vi "camera info.vi"(8 "Disc Number":string, 10 "Camera Name":T1="cam5") -> ()   [LabVIEW 2019]
uses:
  <vilib>/userDefined/High Color/IMAQdx.ctl
  <vilib>/vision/driver/NI_Vision_Acquisition_Software.lvlib
  <resource>/objmgr/imaqdx.rc
panel:
  in  "Close":bool
  out "String":string
  out "Temperature State":string
  out "error out":errorcluster
  out "Gain Raw":u32
  out "Exposure Time":u32
  out "Temperature":dbl
  in  "error in":errorcluster
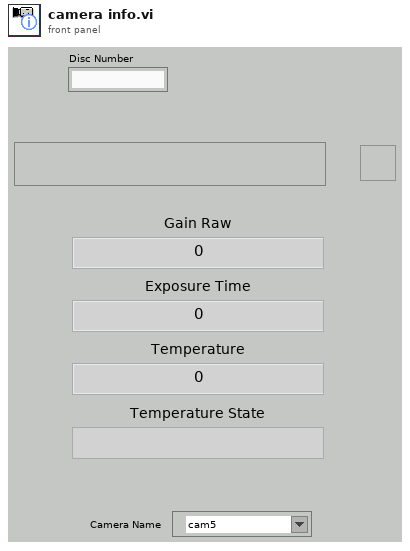
[diagram p1: front panel]
types:
  T1 = typedef "IMAQdx.ctl" = refnum<k21>
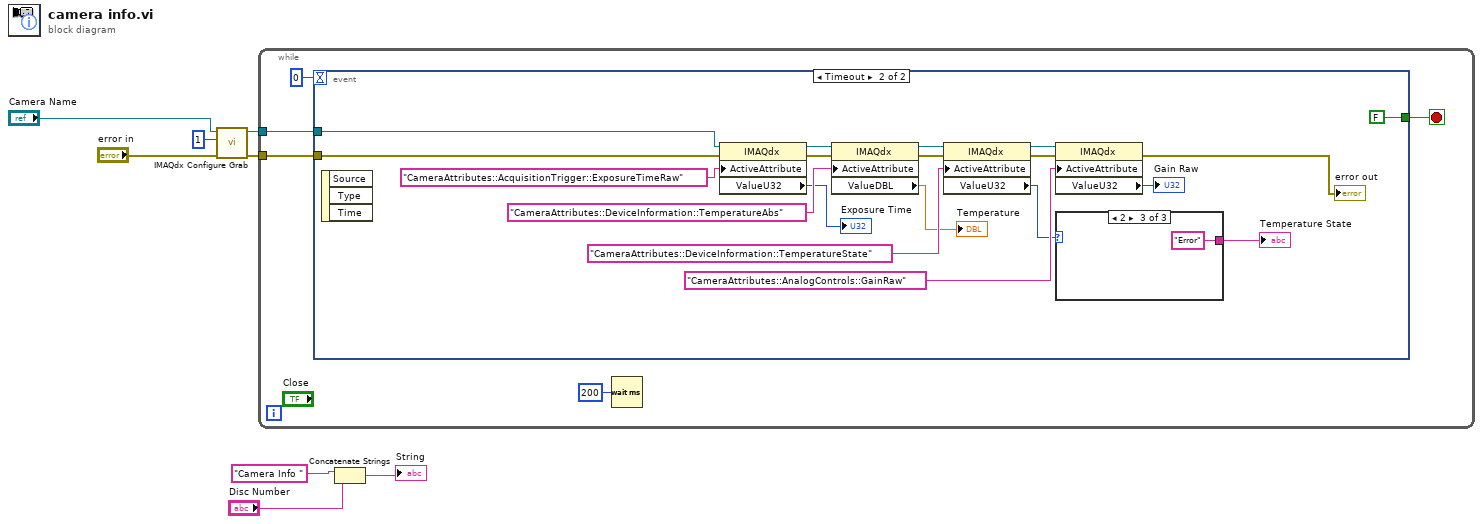
[diagram p0: block diagram]
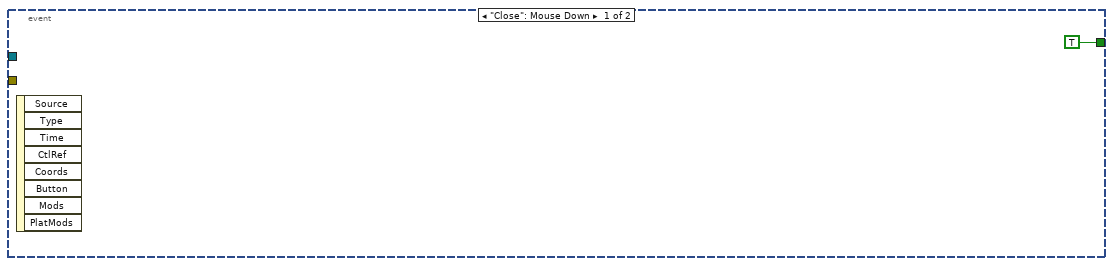
[diagram p2: hidden frame]
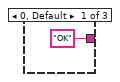
[diagram p3: hidden frame]
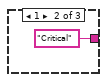
[diagram p4: hidden frame]
diagram:
  n1 = call <vilib>:"IMAQdx Configure Grab.vi"("error in"="error in", "Number of Buffers"=u32 1, "Session In"="Camera Name") -> ("error out"=w6:errorcluster, "Session Out"=w7:T1)  [unwired: 7 in]
  n2 = while {
    tunnel: w7 -> [w13]
    tunnel: w6 -> [w12]
    stop <- w10 stop-if-true
    n3 = event shown="[1] Timeout" {
      selector: _ -> [_ _]
      dyn-events: _ -> [_ _]
      timeout: 0 -> [_ _]
      tunnel: w13 -> [_ w33]
      tunnel: w12 -> [_ w32]
      tunnel: [TRUE FALSE] -> w10
      event "Close": Mouse Down {
        n4 = event-data() -> ()  [unwired: 1 in, 8 out]
      }
      event Timeout {
        n5 = event-data() -> ()  [unwired: 1 in, 3 out]
        n6 = property class="IMAQdx"(reference=w33, error in=w32, "ActiveAttribute"="CameraAttributes::AcquisitionTrigger::ExposureTimeRaw") -> (reference out=w28:T1, error out=w29:errorcluster, "ValueU32"=→"Exposure Time":u32)
        n7 = property class="IMAQdx"(reference=w28, error in=w29, "ActiveAttribute"="CameraAttributes::DeviceInformation::TemperatureAbs") -> (reference out=w27:T1, error out=w26:errorcluster, "ValueDBL"=→"Temperature":dbl)
        n8 = property class="IMAQdx"(reference=w27, error in=w26, "ActiveAttribute"="CameraAttributes::DeviceInformation::TemperatureState") -> (reference out=w24:T1, error out=w23:errorcluster, "ValueU32"=w22:u32)
        n9 = property class="IMAQdx"(reference=w24, error in=w23, "ActiveAttribute"="CameraAttributes::AnalogControls::GainRaw") -> (error out=→"error out":errorcluster, "ValueU32"=→"Gain Raw":u32)  [unwired: 1 out]
        n10 = case shown="2" w22 {
          tunnel: ["OK" ("Temperature State") "Critical" ("Temperature State") "Error" ("Temperature State")] -> w18
          frame 0, Default {
          }
          frame 1 {
          }
          frame 2 {
          }
        }
        "Temperature State" <- w18
      }
    }
    n11 = Wait (ms)(milliseconds to wait=u32 200) -> ()  [unwired: 1 out]
  }
  n12 = Concatenate Strings("Camera Info " ("String"), "Disc Number") -> (→"String":string)
